vi "Write Port.vi"(8 "error in (no error)":errorcluster, 10 "port":u16, 11 "TCP master in":refnum<class "TCP Master.lvclass">) -> (0 "error out":errorcluster, 3 "TCP master out":refnum<class "TCP Master.lvclass">)   [LabVIEW 2020, in "SubVIs.lvlib" / "TCP Master.lvclass"]
doc: "Property accessor for the TCP port."
uses:
  <vilib>/Modbus/subvis/Protocol/TCP/TCP Master/TCP Master.lvclass
  <vilib>/Modbus/subvis/Protocol/TCP/TCP Master/TCP Master.lvclass/TCP Master.ctl
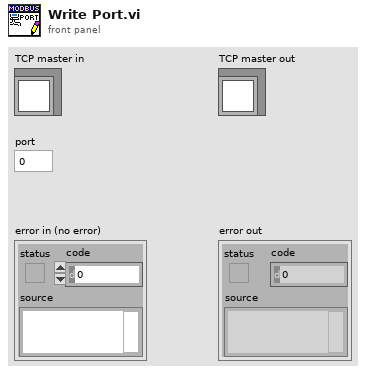
[diagram p1: front panel]
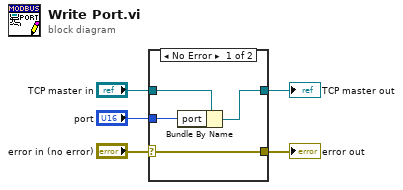
[diagram p0: block diagram]
diagram:
  n1 = case shown="No Error" "error in (no error)" {
    selector: "error in (no error)" -> [w6 w11]
    tunnel: "TCP master in" -> [w9 w10]
    tunnel: [w8 w10] -> w4
    tunnel: "port" -> [w7 _]
    tunnel: [w6 w11] -> w1
    frame No Error {
      n2 = Bundle By Name(cluster=w9, "port"=w7) -> (w8:refnum<class "TCP Master.lvclass">)
    }
    frame Error {
    }
  }
  "error out" <- w1
  "TCP master out" <- w4
